vi "Read Discrete Inputs.vi"(8 "error in (no error)":errorcluster, 9 "number of discrete inputs":u16, 10 "starting address":u16, 11 "Modbus master in":refnum<class "Modbus Master.lvclass">) -> (0 "error out":errorcluster, 2 "discrete input values":bool[](array[boolean]), 3 "Modbus master out":refnum<class "Modbus Master.lvclass">)   [LabVIEW 2021, in "Modbus Master.lvclass"]
doc: "Reads values from contiguous discrete inputs. The maximum number of discrete inputs this VI can read is 2,000."
uses:
  Modbus Master.lvclass
  Modbus Master.lvclass/Modbus Master.ctl
  Modbus Data Unit/Modbus Data Unit.lvclass/Modbus Data Unit.ctl
  Network Protocol/Network Master/Network Master.lvclass/Network Master.ctl
  Master Function Definition/Read Discrete Inputs Request.vi
  Network Protocol/Network Master/Read write Master.vi
  Master Function Definition/Read Discrete Inputs Response.vi
  Modbus Data Unit/Construct PDU.vi
  Utility/Bytes to Bits.vi
  Master Function Definition/Function code mismatch error.vi
  Data Model/Error Generator.vi
  Modbus Data Unit/Deconstruct PDU.vi
  Modbus Data Unit/Modbus Data Unit.lvclass
  Transmission Data Unit/Transmission Data Unit.lvclass
  Network Protocol/Network Master/Network Master.lvclass
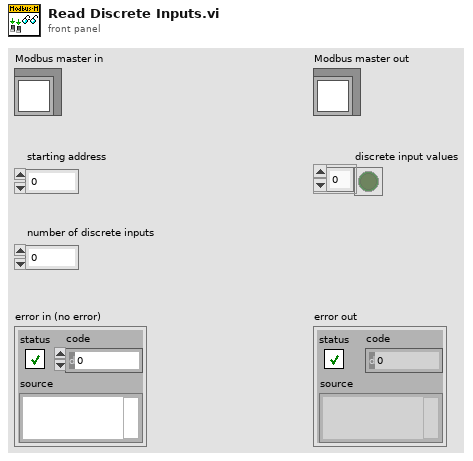
[diagram p1: front panel]
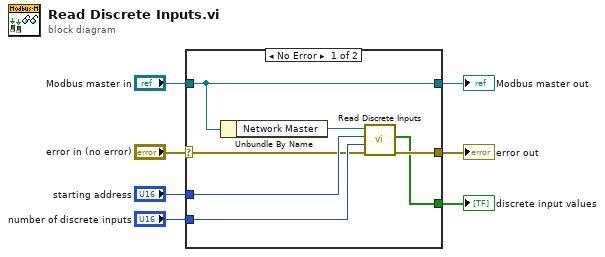
[diagram p0: block diagram]
diagram:
  n1 = case shown="No Error" "error in (no error)" {
    selector: "error in (no error)" -> [w8 w15]
    tunnel: "Modbus master in" -> [w9 w16]
    tunnel: [w9 w16] -> w6
    tunnel: [w14 w15] -> w5
    tunnel: [w11 _] -> w3
    tunnel: "number of discrete inputs" -> [w12 _]
    tunnel: "starting address" -> [w13 _]
    frame No Error {
      n2 = Unbundle By Name(w9) -> ("Network Master"=w10:refnum<class "Network Master.lvclass">)
      n3 = call "Read Discrete Inputs.vi"("error in (no error)"=w8, "number of discrete inputs"=w12, "starting address"=w13, "Modbus master in"=w10) -> ("error out"=w14:errorcluster, "discrete input values"=w11:bool[])  [unwired: 5 in, 1 out]
    }
    frame Error {
    }
  }
  "error out" <- w5
  "Modbus master out" <- w6
  "discrete input values" <- w3
